vi "Query (static).vi"(6 "timeout in ms (5000)":i32=5000, 8 "error in (no error)":errorcluster, 10 "Message":refnum<class "MSG.lvclass">, 11 "MSR Parent":refnum<class "Send.lvclass">) -> (0 "error out":errorcluster, 2 "Reply":refnum<class "MSG.lvclass">, 3 "MSR Parent":refnum<class "Send.lvclass">)   [LabVIEW 2011, in "Messenging.lvlib" / "Send.lvclass"]
uses:
  Send.lvclass
  TextVarientMessage/MSG.lvclass
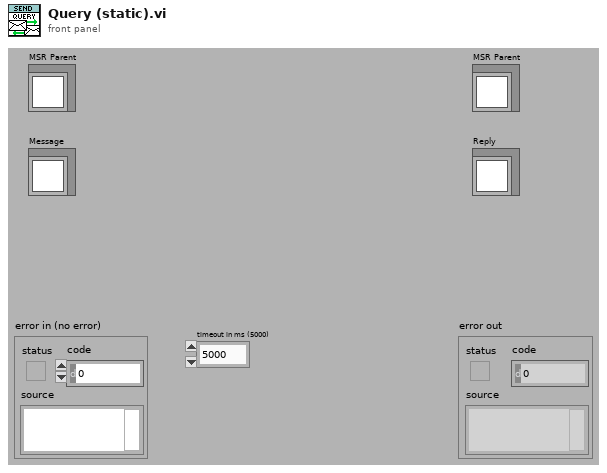
[diagram p1: front panel]
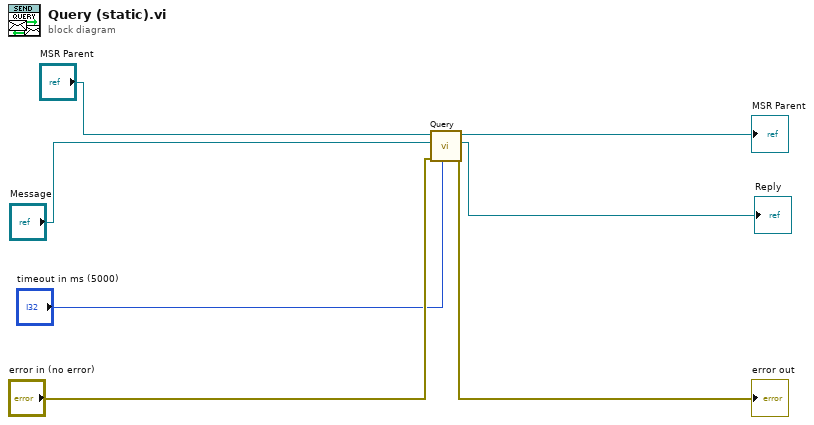
[diagram p0: block diagram]
diagram:
  n1 = call-dynamic "Query.vi"("timeout in ms (5000)"="timeout in ms (5000)", "error in (no error)"="error in (no error)", "Message"="Message", "MSR Parent"="MSR Parent") -> ("error out"=→"error out":errorcluster, "Reply"=→"Reply":refnum<class "MSG.lvclass">, "MSR Parent"=→"MSR Parent":refnum<class "Send.lvclass">)  [unwired: 5 out]
